vi "Parameters_Get_Stop.vi"(11 "Parameters":dbl[](array[numeric])) -> (3 "Stop Mode":i32(ring)=11599968 items=["Decelerate"=11599968, "Immediate"=11599969, "Disable Drive"=11599970])   [LabVIEW 2017, in "WordManipulationLibrary.lvlib"]
uses:
  WordManipulationLibrary.lvlib
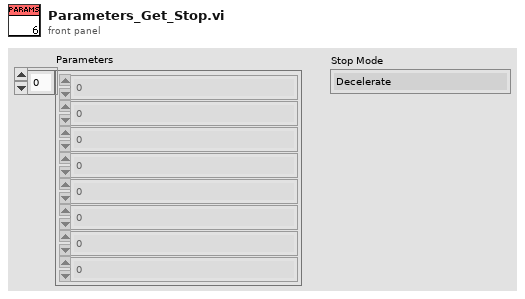
[diagram p1: front panel]
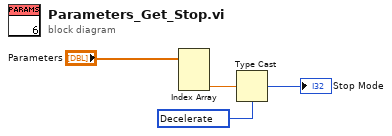
[diagram p0: block diagram]
diagram:
  w2 = 11599968 items=["Decelerate"=11599968, "Immediate"=11599969, "Disable Drive"=11599970] ("Stop Mode")
  n1 = Index Array(array="Parameters") -> (element #3=w3:dbl)  [unwired: 3 in, 2 out]
  n2 = Type Cast(type=w2, x=w3) -> (*(type *) &x=→"Stop Mode":i32)
